vi "VIDM_Main.vi"() -> ()   [LabVIEW 2016]
panel:
  in  "Load":bool
  in  "stop":bool
  in  "Source Folder":path=path "C:/Users/lfbr/Documents/AVERNA-PROJECTS/Av - Training/Labview/LV - RS232 Drivers"
  in  "Write":bool
  in  "Read":bool
  in  "FileList":i32(listbox)
  # "VI Desctiption Manager"
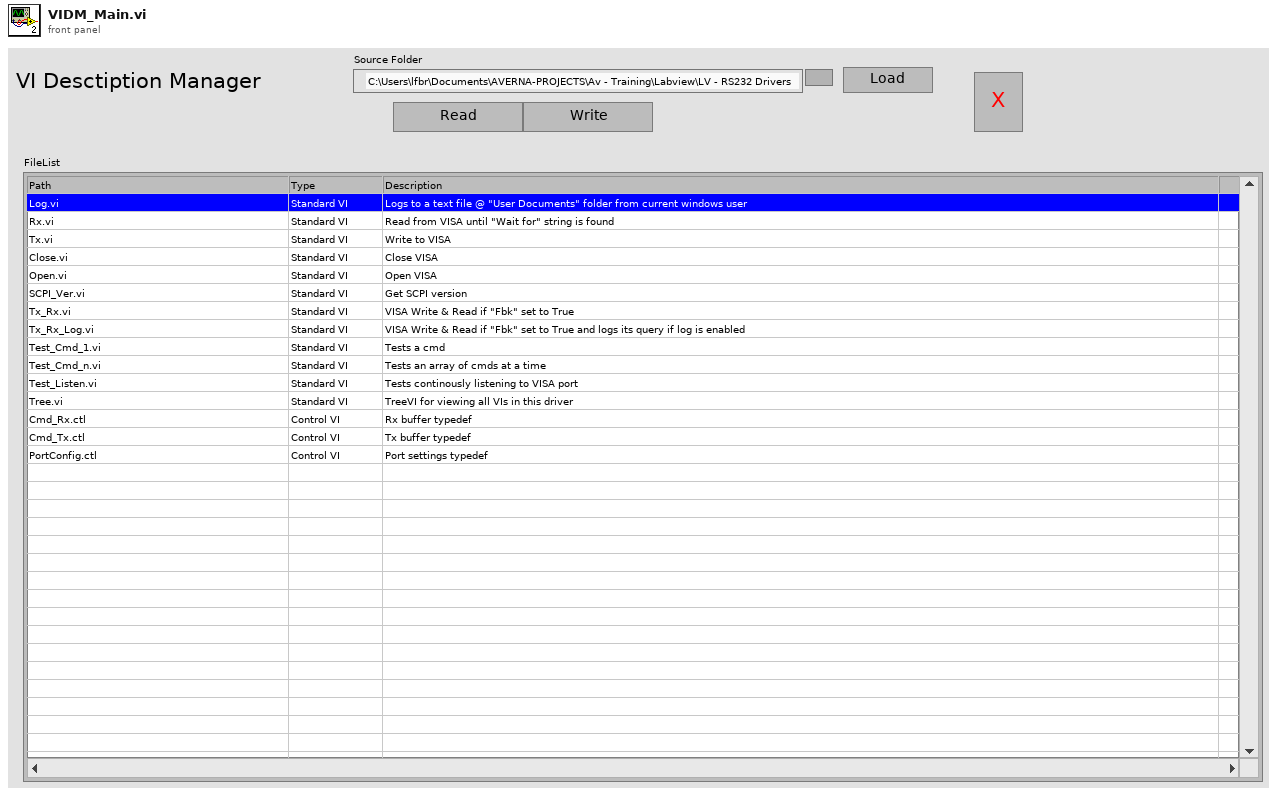
[diagram p1: front panel]
types:
  T1 = enum32{"invalid VI type", "Standard VI", "Control VI", "Global VI", "Polymorphic VI", "Configuration VI", "SubSystem", "Facade VI", "Method VI", "Statechart Diagram VI"}
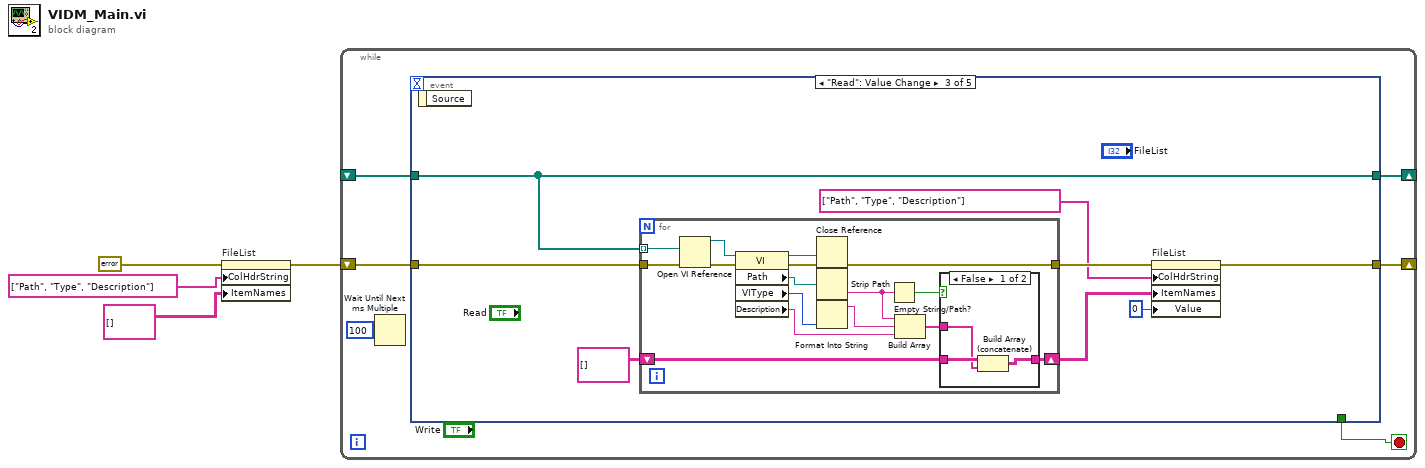
[diagram p0: block diagram]
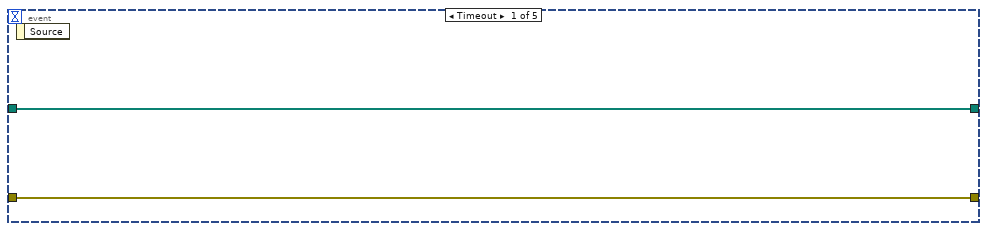
[diagram p2: hidden frame]
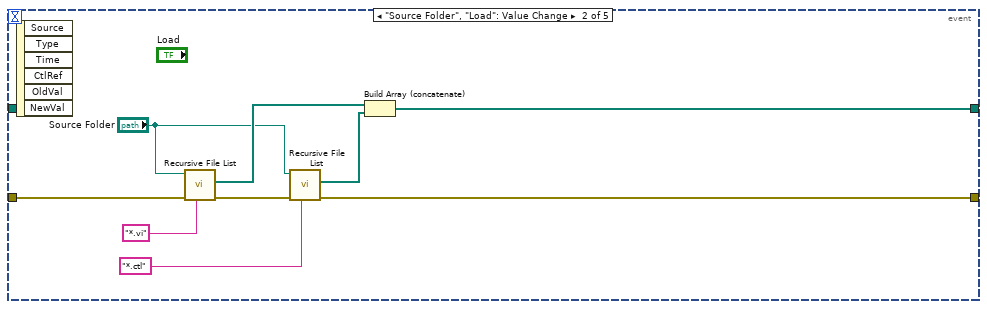
[diagram p3: hidden frame]
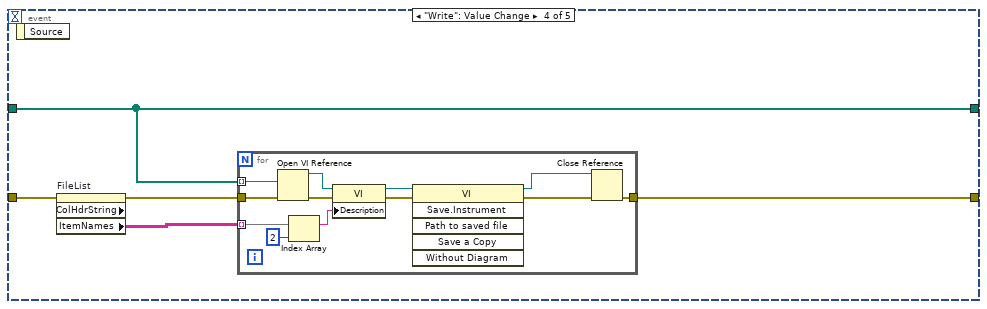
[diagram p5: hidden frame]
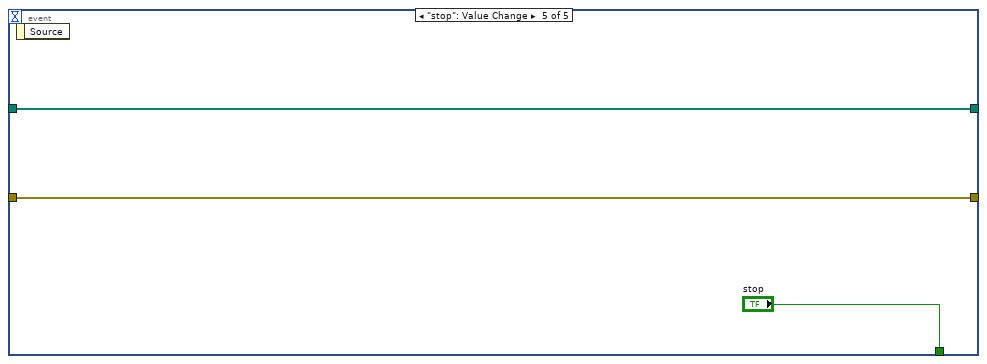
[diagram p6: hidden frame]
diagram:
  n1 = property on="FileList" class="MCListbox (strict)"(error in=errorcluster {"status"=FALSE, "code"=0, "source"=""} ("error in (no error)"), "ColHdrString"=string[] ["Path", "Type", "Description"], "ItemNames"=string[][] []) -> (error out=w3:errorcluster)  [unwired: 1 in, 1 out]
  n2 = while {
    shift-right: [w9] -> _
    shift-left: _ -> [w8]
    shift-right: [w6] -> _
    shift-left: w3 -> [w7]
    stop <- w5 stop-if-true
    n3 = Wait Until Next ms Multiple(millisecond multiple=u32 100 ("millisecond timer value")) -> ()  [unwired: 1 out]
    n4 = event shown="[2] \"Read\": Value Change" {
      selector: _ -> [_ _ _ _ _]
      dyn-events: _ -> [_ _ _ _ _]
      timeout: _ -> [_ _ _ _ _]
      tunnel: [w12 w14 w23 w54 w68] -> w9
      tunnel: w8 -> [w12 _ w23 w54 w68]
      tunnel: w7 -> [w11 w21 w25 w52 w67]
      tunnel: [w11 w13 w24 w53 w67] -> w6
      tunnel: [_ _ _ _ "stop"] -> w5
      event Timeout {
        n5 = event-data() -> ()  [unwired: 1 in, 1 out]
      }
      event "Source Folder", "Load": Value Change {
        n6 = event-data() -> ()  [unwired: 1 in, 6 out]
        n7 = call <vilib>:"Recursive File List.vi"("pattern"="*.vi", "error in (no error)"=w21, "Folder Path"="Source Folder") -> ("error out"=w16:errorcluster, "All Files in Dir"=w19:path[])  [unwired: 4 in, 3 out]
        n8 = call <vilib>:"Recursive File List.vi"("pattern"="*.ctl", "error in (no error)"=w16, "Folder Path"="Source Folder") -> ("error out"=w13:errorcluster, "All Files in Dir"=w18:path[])  [unwired: 4 in, 3 out]
        n9 = Build Array (concatenate)(w19, w18) -> (w14:path[])
      }
      event "Read": Value Change {
        n10 = event-data() -> ()  [unwired: 1 in, 1 out]
        n11 = for {
          shift-right: [w35] -> w28
          shift-left: string[][] [] -> [w34]
          tunnel: [w33] -> w29
          tunnel: w23 -> [w30] mode=indexing
          tunnel: w25 -> [w31]
          n12 = Open VI Reference(vi path=w30, error in (no error)=w31) -> (vi reference=w45:refnum<vi>, error out=w44:errorcluster)  [unwired: 4 in]
          n13 = property class="VI"(reference=w45, error in=w44) -> (reference out=w42:refnum<vi>, error out=w43:errorcluster, "Path"=w41:path, "VIType"=w40:T1, "Description"=w39:string)
          n14 = Close Reference(reference=w42, error in (no error)=w43) -> (error out=w33:errorcluster)
          n15 = Strip Path(path=w41) -> (name=w37:string)  [unwired: 1 out]
          n16 = Format Into String(w40) -> (resulting string=w38:string)  [unwired: 3 in, 1 out]
          n17 = Empty String/Path?(string/path=w37) -> (empty?=w36:bool)
          n18 = Build Array(w37, w38, w39) -> (w32:string[])
          n19 = case shown="False" w36 {
            tunnel: [w47 w49] -> w35
            tunnel: w34 -> [w48 w49]
            tunnel: w32 -> [w46 _]
            frame False {
              n20 = Build Array (concatenate)(w48, w46) -> (w47:string[][])
            }
            frame True {
            }
          }
        }
        n21 = property on="FileList" class="MCListbox (strict)"(error in=w29, "ColHdrString"=string[] ["Path", "Type", "Description"], "ItemNames"=w28, "Value"=0 ("FileList")) -> (error out=w24:errorcluster)  [unwired: 1 in, 1 out]
      }
      event "Write": Value Change {
        n22 = event-data() -> ()  [unwired: 1 in, 1 out]
        n23 = property on="FileList" class="MCListbox (strict)" props=["ColHdrString", "ItemNames"](error in=w52) -> (error out=w51:errorcluster, "ItemNames"=w50:string[][])  [unwired: 1 in, 2 out]
        n24 = for {
          tunnel: [w63] -> w53
          tunnel: w54 -> [w61] mode=indexing
          tunnel: w51 -> [w62]
          tunnel: w50 -> [w60] mode=indexing
          n25 = Open VI Reference(vi path=w61, error in (no error)=w62) -> (vi reference=w66:refnum<vi>, error out=w65:errorcluster)  [unwired: 4 in]
          n26 = Index Array(array=w60, index=2) -> (element=w59:string)
          n27 = property class="VI"(reference=w66, error in=w65, "Description"=w59) -> (reference out=w56:refnum<vi>, error out=w64:errorcluster)
          n28 = invoke class="VI" method="Save.Instrument"(reference=w56, error in=w64) -> (reference out=w55:refnum<vi>, error out=w57:errorcluster)  [unwired: 4 in, 4 out]
          n29 = Close Reference(reference=w55, error in (no error)=w57) -> (error out=w63:errorcluster)
        }
      }
      event "stop": Value Change {
        n30 = event-data() -> ()  [unwired: 1 in, 1 out]
      }
    }
  }
